vi "GetTelemetryUpdateDataSGLConstant.vi"() -> (3 "TelemetryUpdateDataSGL":T1={"Mode"=enum."=", "Field"=enum."InclinometerErrorCode", "Data"=0.0})   [LabVIEW 2018]
uses:
  TelemetryUpdateDataSGL.ctl
  TelemetryUpdateModes.ctl
  TelemetryFields.ctl
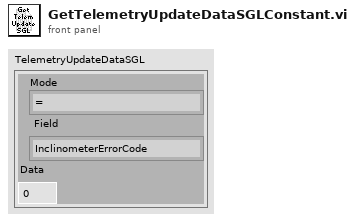
[diagram p1: front panel]
types:
  T1 = typedef "TelemetryUpdateDataSGL.ctl" = cluster{"Mode":T2, "Field":T3, "Data":sgl}
  T2 = typedef "TelemetryUpdateModes.ctl" = enum8{"=", "+", "-", "|"}
  T3 = typedef "TelemetryFields.ctl" = enum16{"None", "InclinometerTxBytes", "InclinometerRxBytes", "InclinometerTxFrames", "InclinometerRxFrames", "InclinometerErrorTimestamp", "InclinometerErrorCode", "InclinometerSampleTimestamp", "InclinometerAngleRaw", "DisplacementTxBytes", "DisplacementRxBytes", "DisplacementTxFrames", "DisplacementRxFrames", "DisplacementErrorTimestamp", "DisplacementErrorCode", "DisplacementSampleTimestamp", "DisplacementRaw1", "DisplacementRaw2", "DisplacementRaw3", "DisplacementRaw4", "DisplacementRaw5", "DisplacementRaw6", "DisplacementRaw7", "DisplacementRaw8", "AccelerometerSampleCount", "AccelerometerSampleTimestamp", "AccelerometerRaw1", "AccelerometerRaw2", "AccelerometerRaw3", "AccelerometerRaw4", "AccelerometerRaw5", "AccelerometerRaw6", "AccelerometerRaw7", "AccelerometerRaw8", "GyroTxBytes", "GyroRxBytes", "GyroTxFrames", "GyroRxFrames", "GyroErrorTimestamp", "GyroErrorCode", "GyroSampleTimestamp", "GyroRawX", "GyroRawY", "GyroRawZ", "GyroStatus", "GyroSequenceNumber", "GyroTemperature", "GyroBITTimestamp", "GyroBIT0", "GyroBIT1", "GyroBIT2", "GyroBIT3", "GyroBIT4", "GyroBIT5", "GyroBIT6", "GyroBIT7", "DigitalInputSampleCount", "DigitalInputTimestamp", "DigitalInputStates", "DigitalOutputSampleCount", "DigitalOutputTimestamp", "DigitalOutputStates", "PowerSupplySampleCount", "PowerSupplyTimestamp", "PowerSupplyStates", "Modbus1ErrorFlags", "Modbus1TxByteCount", "Modbus1TxFrameCount", "Modbus1RxByteCount", "Modbus1RxFrameCount", "Modbus2ErrorFlags", "Modbus2TxByteCount", "Modbus2TxFrameCount", "Modbus2RxByteCount", "Modbus2RxFrameCount", "Modbus3ErrorFlags", "Modbus3TxByteCount", "Modbus3TxFrameCount", "Modbus3RxByteCount", "Modbus3RxFrameCount", "Modbus4ErrorFlags", "Modbus4TxByteCount", "Modbus4TxFrameCount", "Modbus4RxByteCount", "Modbus4RxFrameCount"}
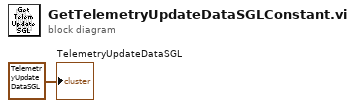
[diagram p0: block diagram]
diagram:
  "TelemetryUpdateDataSGL" <- T1 {"Mode"=enum."=", "Field"=enum."InclinometerErrorCode", "Data"=0.0} ("TelemetryUpdateDataSGL")
